vi "G-signal.vi"() -> ()   [LabVIEW 2014]
panel:
  in  "测试总数":dbl
  in  "合格数":dbl
  out "G halt":bool
  out "G stop":bool
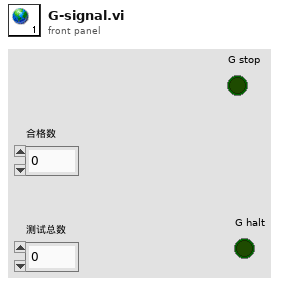
[diagram p1: front panel]
diagram:
